vi "svm_predict_probabilities.vi"(8 "error in (no error)":errorcluster, 10 "X":T1[](array[typedef])=[{"index"=0, "value"=0.0}], 11 "Model":T2) -> (0 "error out":errorcluster, 2 "Probability estimates":dbl[](array[numeric]), 3 "Predicted label":dbl)   [LabVIEW 2015]
doc: "This function does classification or regression on a test vector x given a model with probability information.\n\nFor a classification model with probability information, this function gives nr_class probability estimates in the output array probability estimates."
uses:
  Controls/svm_model.ctl
  Controls/svm_parameter.ctl
  Controls/svm_type.ctl
  Controls/svm_kernel_type.ctl
  Controls/svm_node.ctl
  bin/LabVIEW-libsvm.so
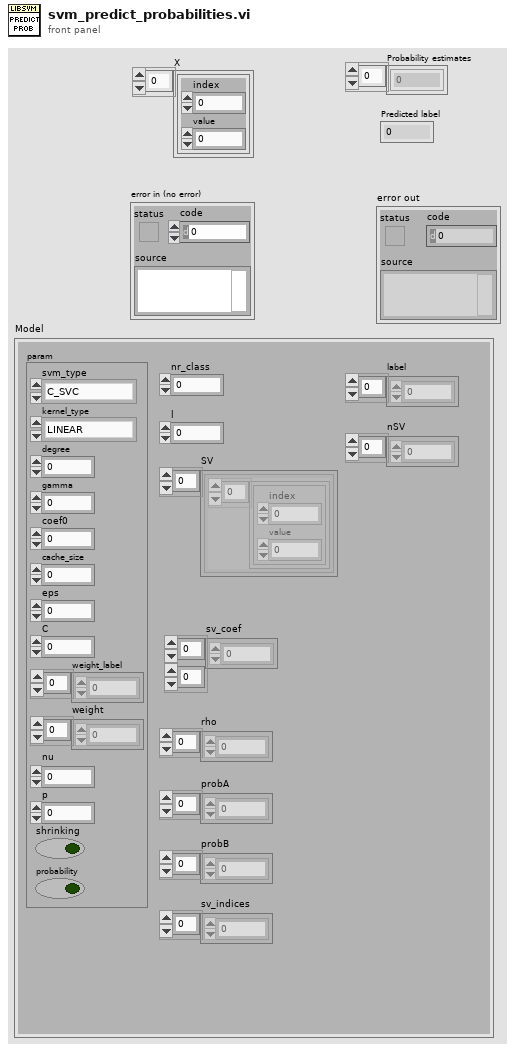
[diagram p1: front panel]
types:
  T1 = typedef "svm_node.ctl" = cluster{"index":i32, "value":dbl}
  T2 = typedef "svm_model.ctl" = cluster{"param":T3, "nr_class":i32, "l":i32, "SV":cluster{"Array":T1[]}[], "sv_coef":dbl[][], "rho":dbl[], "probA":dbl[], "probB":dbl[], "sv_indices":i32[], "label":i32[], "nSV":i32[]}
  T3 = typedef "svm_parameter.ctl" = cluster{"svm_type":T4, "kernel_type":T5, "degree":i32, "gamma":dbl, "coef0":dbl, "cache_size":dbl, "eps":dbl, "C":dbl, "weight_label":i32[], "weight":dbl[], "nu":dbl, "p":dbl, "shrinking":bool, "probability":bool}
  T4 = typedef "svm_type.ctl" = enum32{"C_SVC", "NU_SVC", "ONE_CLASS", "EPSILON_SVR", "NU_SVR"}
  T5 = typedef "svm_kernel_type.ctl" = enum32{"LINEAR", "POLY", "RBF", "SIGMOID", "PRECOMPUTED"}
  T6 = typedef "svm_node_padded.ctl" = cluster{"index":i32, "padding":i32, "value":dbl}
  T7 = typedef "svm_model_padded.ctl" = cluster{"param":T3, "nr_class":i32, "l":i32, "SV":cluster{"Array":T6[]}[], "sv_coef":dbl[][], "rho":dbl[], "probA":dbl[], "probB":dbl[], "sv_indices":i32[], "label":i32[], "nSV":i32[]}
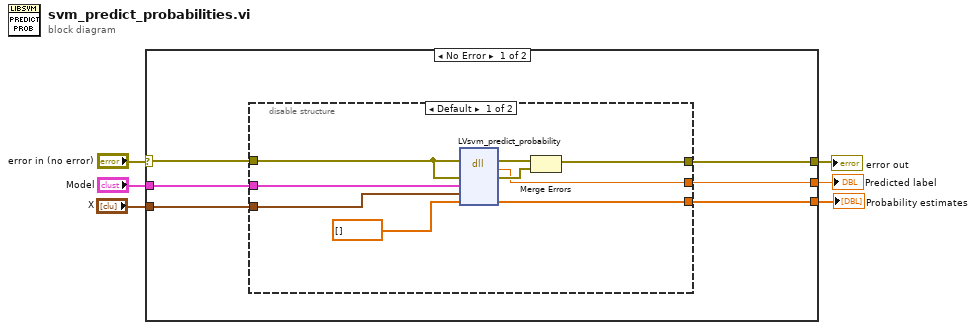
[diagram p0: block diagram]
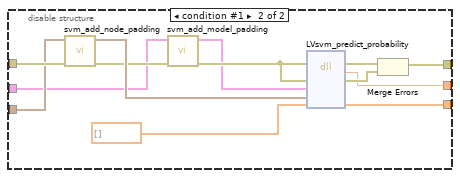
[diagram p2: hidden frame]
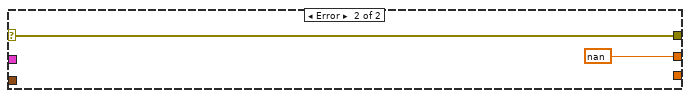
[diagram p3: hidden frame]
diagram:
  n1 = case shown="No Error" "error in (no error)" {
    selector: "error in (no error)" -> [w12 w36]
    tunnel: [w11 w36] -> w6
    tunnel: "Model" -> [w10 _]
    tunnel: "X" -> [w9 _]
    tunnel: [w8 nan ("predicted label")] -> w2
    tunnel: [w7 _] -> w1
    frame No Error {
      n2 = disable-structure shown="Default" {
        disable-tunnel: w12 -> [w21 w28]
        disable-tunnel: [w18 w32] -> w11
        disable-tunnel: w10 -> [w17 w23]
        disable-tunnel: w9 -> [w16 w27]
        disable-tunnel: [w15 w31] -> w8
        disable-tunnel: [w13 w29] -> w7
        frame condition #0 (active) {
          n3 = dll-call lib="home/os/dev/LabVIEW-libsvm/LabVIEW/bin/LabVIEW-libsvm.*" fn="LVsvm_predict_probability"(error in=w21, "lvErr"=w21, "model_in"=w17, "x_in"=w16, "prob_estimates_out"=dbl[] [] ("dec_values_out")) -> (error out=w20:errorcluster, "predicted label"=w15:dbl, "lvErr"=w19:errorcluster, "prob_estimates_out"=w13:dbl[])  [unwired: 4 in, 1 out]
          n4 = Merge Errors(w20, w19) -> (w18:errorcluster)
        }
        frame condition #1 {
          n5 = call "svm_add_node_padding.vi"("error in (no error)"=w28, "Nodes"=w27) -> ("error out"=w25:errorcluster, "Padded nodes"=w26:T6[])  [unwired: 8 in]
          n6 = call "svm_add_model_padding.vi"("error in (no error)"=w25, "Model"=w23) -> ("error out"=w24:errorcluster, "Padded model"=w22:T7)  [unwired: 8 in]
          n7 = dll-call lib="home/os/dev/LabVIEW-libsvm/LabVIEW/bin/LabVIEW-libsvm.*" fn="LVsvm_predict_probability"(error in=w24, "lvErr"=w24, "model_in"=w22, "x_in"=w26, "prob_estimates_out"=dbl[] [] ("dec_values_out")) -> (error out=w34:errorcluster, "predicted label"=w31:dbl, "lvErr"=w33:errorcluster, "prob_estimates_out"=w29:dbl[])  [unwired: 4 in, 1 out]
          n8 = Merge Errors(w34, w33) -> (w32:errorcluster)
        }
      }
    }
    frame Error {
    }
  }
  "error out" <- w6
  "Predicted label" <- w2
  "Probability estimates" <- w1
